vi "Fit.I-V.subvi.vi"(0 "y":dbl[](array[numeric]), 1 "x":dbl[](array[numeric]), 2 "Name      Guess     Fit?":T1={"parameter"="Is(A)", "guess"=0.01, "Fit?"=TRUE} {"guess" min=0.1 step=0.1}, 3 "Parameter Name      Parameter Guess        Fit?":T1={"parameter"="Vfl(V)", "guess"=-10.0, "Fit?"=TRUE}, 4 "Parameter Name      Parameter Guess        Fit?":T1={"parameter"="Te(eV)", "guess"=10.0, "Fit?"=TRUE} {"guess" min=0.1}, 5 "reference":refnum<vi>, 9 "set the range by \ncursors?":bool) -> (6 "parameter guess Fit? best fit result":T2(array[cluster])=[{"parameter"="Is(A)", "guess"=0.01, "Fit?"=TRUE, "best fit"=0.01, "result"=0.01}, {"parameter"="Vfl(V)", "guess"=-10.0, "Fit?"=TRUE, "best fit"=-10.0, "result"=-10.0}, {"parameter"="Te(eV)", "guess"=10.0, "Fit?"=TRUE, "best fit"=10.0, "result"=10.0}], 7 "V-I&guess&bestfit":cluster{cdb[]}[](array[cluster]), 8 "ln(I,I-bestfit)":cluster{cdb[]}[](array[cluster]), 10 "error out":errorcluster)   [LabVIEW 2014]
uses:
  <vilib>/gmath/NumericalOptimization/Nonlinear Curve Fit LM.vi
  <vilib>/gmath/NI_Gmath.lvlib
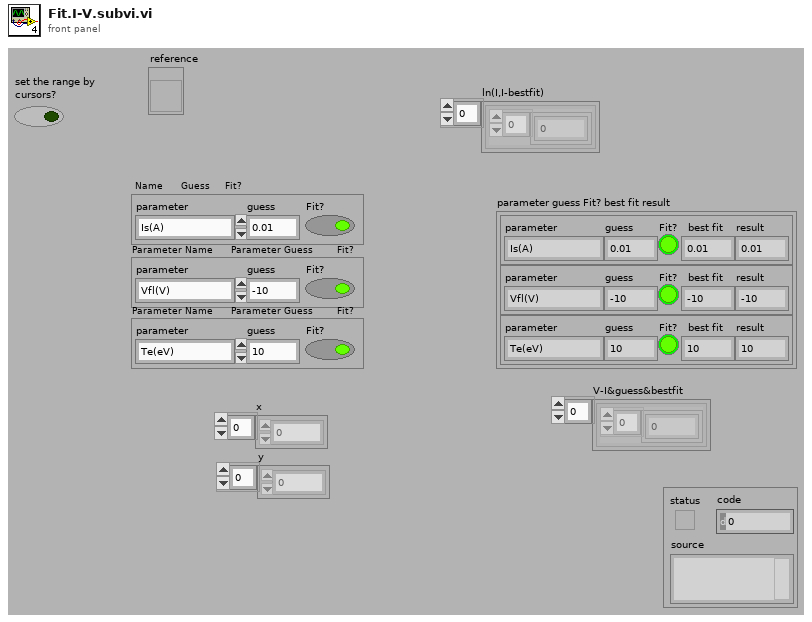
[diagram p1: front panel]
types:
  T1 = cluster{"parameter":string, "guess":dbl, "Fit?":bool}
  T2 = cluster{"parameter":string, "guess":dbl, "Fit?":bool, "best fit":dbl, "result":dbl}[]
  T3 = cluster{"parameter":string, "guess":dbl, "Fit?":bool}[]
  T4 = typedef "LVCursorListTypeDef.ctl" = cluster{"Name":string, "Color":u32, "Style":u8, "Point Style":u8, "Name Visible":bool, "Allow Drag":bool, "Cursor Mode":u32, "Plot":i32, "Index":i32, "Position":cluster{"X":dbl, "Y":dbl}, "X Scale":u32, "Y Scale":u32, "Watch Plots":i32[], "Watch All Plots":bool, "Plot Area":i32, "Label Offset":cluster{"X":dbl, "Y":dbl}}[]
  T5 = cluster{"Name":string, "Color":u32, "Style":u8, "Point Style":u8, "Name Visible":bool, "Allow Drag":bool, "Cursor Mode":u32, "Plot":i32, "Index":i32, "Position":cluster{"X":dbl, "Y":dbl}, "X Scale":u32, "Y Scale":u32, "Watch Plots":i32[], "Watch All Plots":bool, "Plot Area":i32, "Label Offset":cluster{"X":dbl, "Y":dbl}}
  T6 = cluster{"parameter":string, "guess":dbl, "Fit?":bool, "best fit":dbl, "result":dbl}
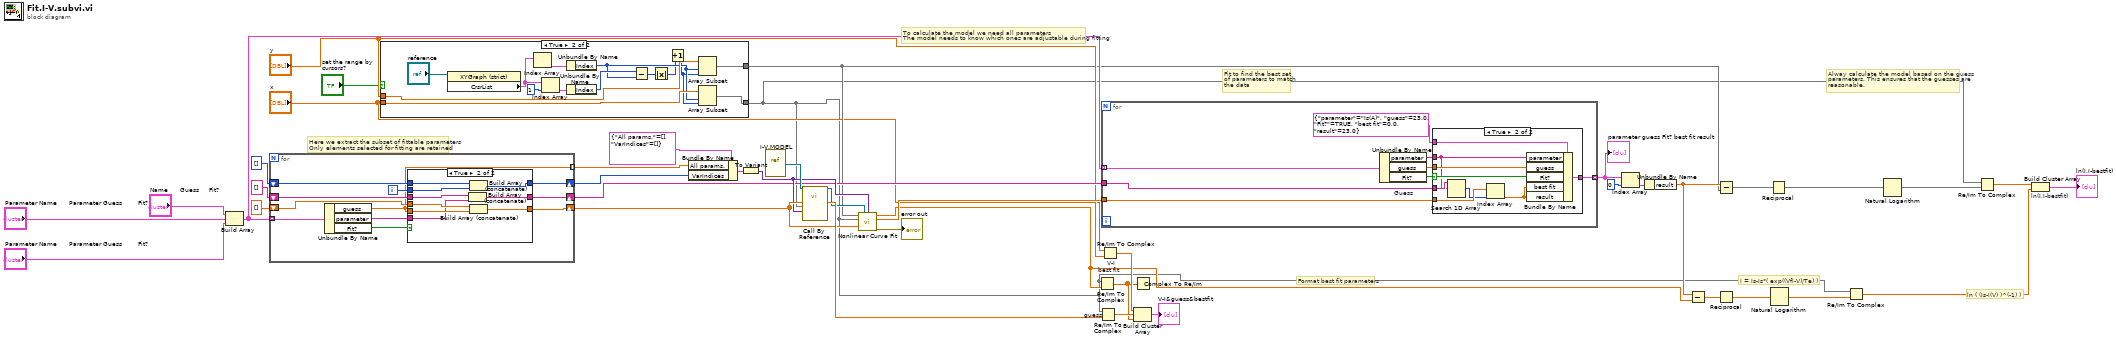
[diagram p0: block diagram]
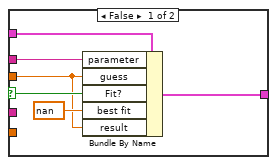
[diagram p3: hidden frame]
diagram:
  # "I = Is-Is*( exp((Vfl-V)/Te) )"
  # "ln ( (Is-I(V) )^(-1) )"
  # "Fit to find the best set\nof parameters to match\nthe data"
  # "Format best fit parameters"
  # "Alway calculate the model based on the guess\nparameters. This ensures that the guesses are\nreasonable."
  # "To calculate the model we need all parameters\nThe model needs to know which ones are adjustable during fitting"
  # "Here we extract the subset of fittable parameters\nOnly elements selected for fitting are retained"
  n1 = Build Array("Name      Guess     Fit?", "Parameter Name      Parameter Guess        Fit?", "Parameter Name      Parameter Guess        Fit?") -> (w23:T3)
  n2 = for {
    shift-right: [w53] -> w35
    shift-left: dbl[] [] -> [w52]
    tunnel: w23 -> [w51] mode=indexing
    tunnel: [w44] -> w33 mode=indexing
    shift-right: [w49] -> w32
    shift-left: i32[] [] -> [w48]
    shift-right: [w45] -> w28
    shift-left: string[] [] -> [w46]
    i -> [w47]
    n3 = Unbundle By Name(w51) -> ("guess"=w44:dbl, "parameter"=w43:string, "Fit?"=w50:bool)
    n4 = case shown="True" w50 {
      tunnel: [w56 w64] -> w53
      tunnel: w52 -> [w56 w65]
      tunnel: w44 -> [_ w63]
      tunnel: [w55 w62] -> w49
      tunnel: w48 -> [w55 w61]
      tunnel: w47 -> [_ w60]
      tunnel: [w54 w58] -> w45
      tunnel: w46 -> [w54 w59]
      tunnel: w43 -> [_ w57]
      frame False {
      }
      frame True {
        n5 = Build Array (concatenate)(w59, w57) -> (w58:string[])
        n6 = Build Array (concatenate)(w61, w60) -> (w62:i32[])
        n7 = Build Array (concatenate)(w65, w63) -> (w64:dbl[])
      }
    }
  }
  n8 = case shown="True" "set the range by \ncursors?" {
    tunnel: [w67 w71] -> w1
    tunnel: "x" -> [w67 w73]
    tunnel: [w66 w74] -> w4
    tunnel: "y" -> [w66 w79]
    frame False {
    }
    frame True {
      n9 = property on="Property Node" class="XYGraph (strict)"(reference="reference") -> ("CrsrList"=w78:T4)  [unwired: 1 in, 2 out]
      n10 = Index Array(array=w78) -> (element=w77:T5)  [unwired: 1 in]
      n11 = Index Array(array=w78, index=1) -> (element=w81:T5)
      n12 = Unbundle By Name(w77) -> ("Index"=w72:i32)
      n13 = Unbundle By Name(w81) -> ("Index"=w75:i32)
      n14 = Subtract(x=w75, y=w72) -> (x-y=w70:i32)
      n15 = Absolute Value(x=w70) -> (abs(x)=w69:i32)
      n16 = Increment(x=w69) -> (x+1=w68:i32)
      n17 = Array Subset(array=w79, index=w72, length=w68) -> (w74:dbl[])
      n18 = Array Subset(array=w73, index=w72, length=w68) -> (w71:dbl[])
    }
  }
  n19 = Bundle By Name(cluster=cluster{"All params.":dbl[], "VarIndices":i32[]} {"All params."=[], "VarIndices"=[]}, "All params."=w33, "VarIndices"=w32) -> (w36:cluster{"All params.":dbl[], "VarIndices":i32[]})
  n20 = To Variant(anything=w36) -> (Variant=w30:variant)
  n21 = vi-ref "I-V.MODEL.vi"() -> (w42:refnum<vi>)
  n22 = call-by-ref "Call By Reference"(reference=w42, "data"=w30, "frequency"=w1, "tau"=w35) -> (reference out=w37:refnum<vi>, "Phase"=w39:dbl[])  [unwired: 2 in, 3 out]
  n23 = call-poly <vilib>:"Nonlinear Curve Fit.vi"("Y"=w4, "f(x,a)"=w37, "data"=w30, "X"=w1, "initial parameters"=w35) -> ("best nonlinear fit"=w3:dbl[], "best fit parameters"=w27:dbl[], "error out"=→"error out":errorcluster)  [unwired: 5 in, 3 out]
  n24 = Re/Im To Complex "best fit"(1:w3, 2:w1) -> (0:w11:cdb[])
  n25 = Re/Im To Complex "guess"(1:w39, 2:w1) -> (0:w22:cdb[])
  n26 = for {
    tunnel: w23 -> [w89] mode=indexing
    tunnel: w28 -> [w85]
    tunnel: w27 -> [w84]
    tunnel: [w83] -> w13 mode=indexing
    n27 = Unbundle By Name "Guess"(w89) -> ("parameter"=w88:string, "guess"=w86:dbl, "Fit?"=w87:bool)
    n28 = case shown="True" w87 {
      selector: w87 -> [w95 w103]
      tunnel: T6 {"parameter"="Is(A)", "guess"=23.0, "Fit?"=TRUE, "best fit"=0.0, "result"=23.0} ("ParameterSelect") -> [w94 w104]
      tunnel: w88 -> [w91 w97]
      tunnel: w86 -> [w90 w102]
      tunnel: w85 -> [_ w101]
      tunnel: w84 -> [_ w100]
      tunnel: [w93 w98] -> w83
      frame False {
        n29 = Bundle By Name(cluster=w94, "parameter"=w91, "guess"=w90, "Fit?"=w95, "best fit"=nan, "result"=w90) -> (w93:T6)
      }
      frame True {
        n30 = Search 1D Array(1D array=w101, element=w97) -> (index of element=w99:i32)  [unwired: 1 in]
        n31 = Index Array(array=w100, index=w99) -> (element=w96:dbl)
        n32 = Bundle By Name(cluster=w104, "parameter"=w97, "guess"=w102, "Fit?"=w103, "best fit"=w96, "result"=w96) -> (w98:T6)
      }
    }
  }
  "parameter guess Fit? best fit result" <- w13
  n33 = Re/Im To Complex "V-I"(1:"y", 2:"x") -> (0:w12:cdb[])
  n34 = Build Cluster Array(w12, w22, w11) -> (→"V-I&guess&bestfit":cluster{cdb[]}[])
  n35 = Complex To Re/Im(x + iy=w11) -> ()  [unwired: 2 out]
  n36 = Index Array(array=w13, index=0) -> (element=w17:T6)
  n37 = Unbundle By Name(w17) -> ("result"=w7:dbl)
  n38 = Subtract(x=w7, y=w3) -> (x-y=w15:dbl[])
  n39 = Subtract(x=w7, y=w4) -> (x-y=w20:dbl[])
  n40 = Reciprocal(x=w15) -> (1/x=w14:dbl[])
  n41 = Reciprocal(x=w20) -> (1/x=w19:dbl[])
  n42 = Natural Logarithm(1:w14) -> (0:w16:dbl[])
  n43 = Re/Im To Complex(1:w16, 2:w1) -> (0:w8:cdb[])
  n44 = Natural Logarithm(1:w19) -> (0:w21:dbl[])
  n45 = Re/Im To Complex(1:w21, 2:w1) -> (0:w9:cdb[])
  n46 = Build Cluster Array "ln(I,I-bestfit)"(w9, w8) -> (→"ln(I,I-bestfit)":cluster{cdb[]}[])
